vi "332meas.vi"() -> (1 "332 Temp [K]":dbl format="%.3f", 2 "332 Temp Setpoint [K]":dbl)   [LabVIEW 2012]
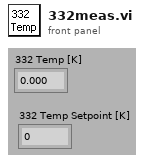
[diagram p1: front panel]
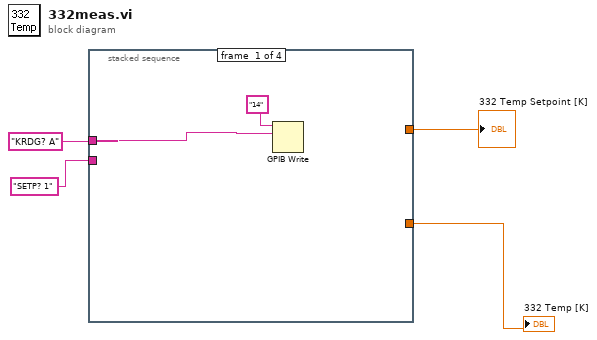
[diagram p0: block diagram]
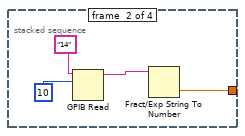
[diagram p2: hidden frame]
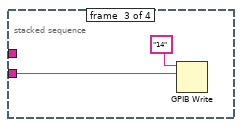
[diagram p3: hidden frame]
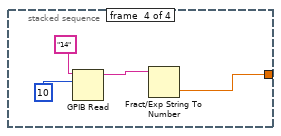
[diagram p4: hidden frame]
diagram:
  n1 = stacked-sequence {
    tunnel: [_ w9 _ _] -> w4
    tunnel: "KRDG? A" -> [w5 _ _ _]
    tunnel: "SETP? 1" ("data") -> [_ _ w11 _]
    tunnel: [_ _ _ w13] -> w1
    frame #0 {
      n2 = GPIB Write(0:"14", 1:w5) -> ()  [unwired: 3 in, 2 out]
    }
    frame #1 {
      n3 = GPIB Read(0:"14", 1:10) -> (5:w10:string)  [unwired: 3 in, 2 out]
      n4 = Fract/Exp String To Number(string=w10) -> (number=w9:dbl)  [unwired: 3 in, 1 out]
    }
    frame #2 {
      n5 = GPIB Write(0:"14", 1:w11) -> ()  [unwired: 3 in, 2 out]
    }
    frame #3 {
      n6 = GPIB Read(0:"14", 1:10) -> (5:w14:string)  [unwired: 3 in, 2 out]
      n7 = Fract/Exp String To Number(string=w14) -> (number=w13:dbl)  [unwired: 3 in, 1 out]
    }
  }
  "332 Temp [K]" <- w4
  "332 Temp Setpoint [K]" <- w1
